vi "CBR_Player.vi"() -> ()   [LabVIEW 2012]
panel:
  out "Tiny Lines":string[](array[string])
  out "BotSpeak":string
  out "ComType":T1(ring)
  out "Reply":string
  out "error out":errorcluster
  out "text":string
  in  "Vireo":path=path "/Kim/Users/crogers/Documents/LabVIEW Data/LVVIAGenerated/Demo1.vi  2013-12-18 14-09-36.via"
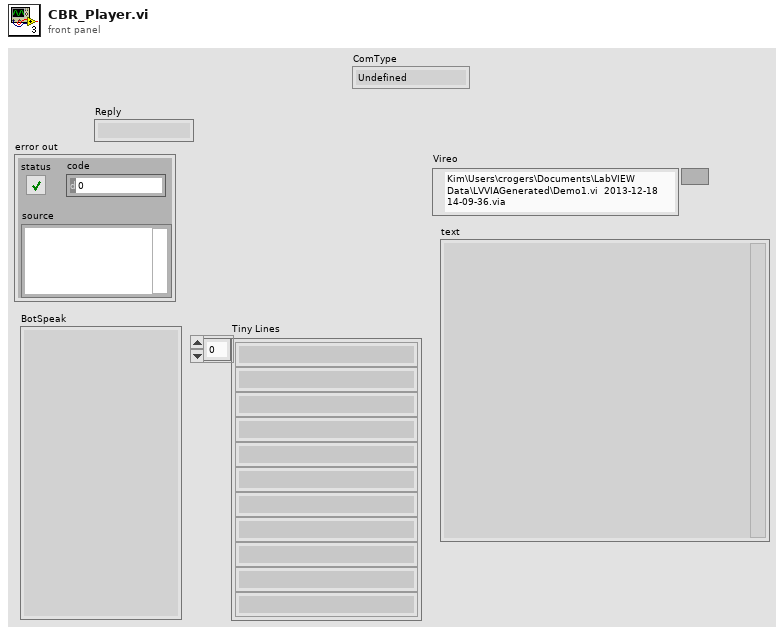
[diagram p1: front panel]
types:
  T1 = enum16{"Undefined", "HTTP", "Serial", "TCPIP", "Console"}
  T2 = typedef "BotSpeak_Control.ctl" = cluster{"Address":string, "Reply EOF":string, "Hardware":string, "Retries":i8, "Timeout":i32, "Open?":bool}
  T3 = typedef "BotSpeak.HardwareSpecs.ctl" = cluster{"Hardware Name":string, "Hardware URL":string, "ComType":enum16{"Undefined", "HTTP", "Serial", "TCPIP", "Console"}, "TCP Port":i32, "DefaultAddress":string, "Retries":i32, "Translate":enum16{"None", "Tiny", "URAPI"}, "MaxScriptSize":i32, "MaxVarNumber":i32, "StartupWait":i32, "Patience":i32, "Startup Patience":i32, "Hardware Help":string, "Com Protocol":string, "Translator":cluster{"BotSpeak CMD":string, "CMD out":string}[], "Init Code":string, "Variable Format":enum16{"INT", "FLOAT", "FIXED"}, "username":string, "password":string}
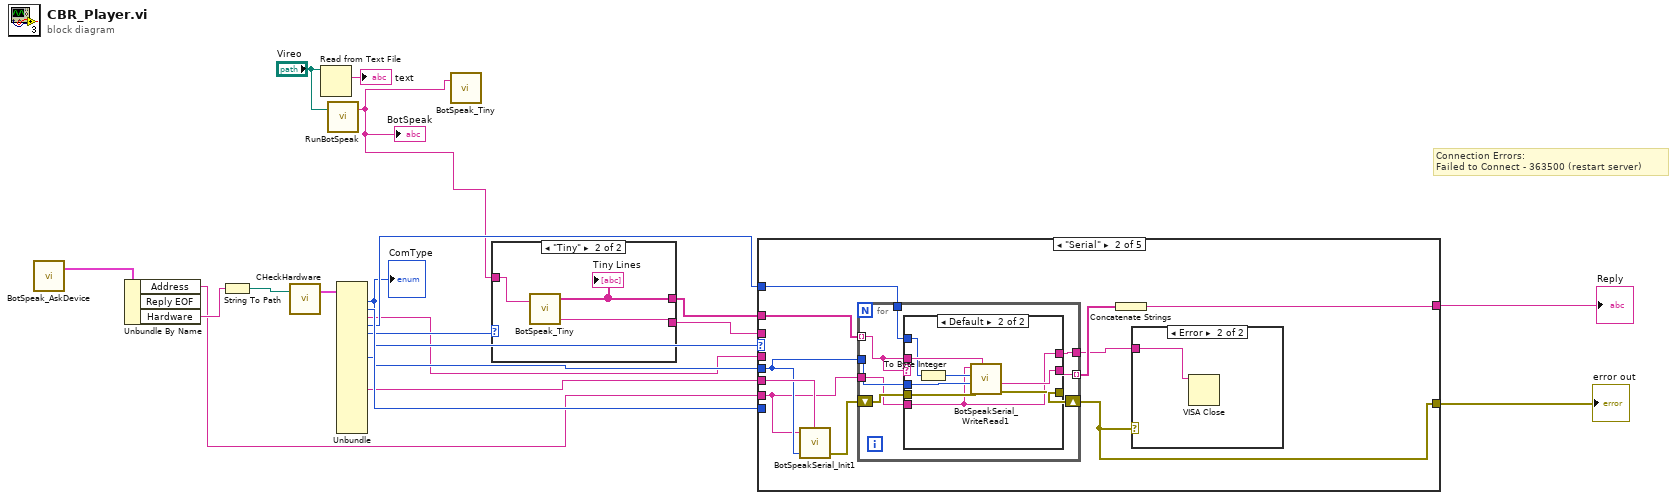
[diagram p0: block diagram]
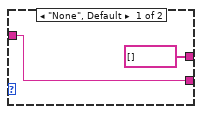
[diagram p2: hidden frame]
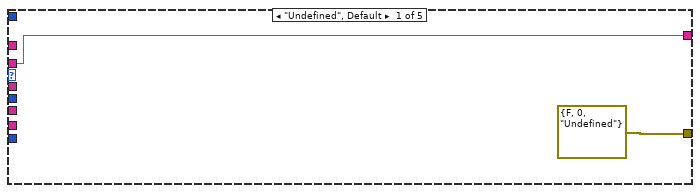
[diagram p3: hidden frame]
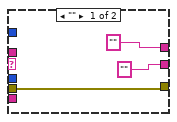
[diagram p4: hidden frame]
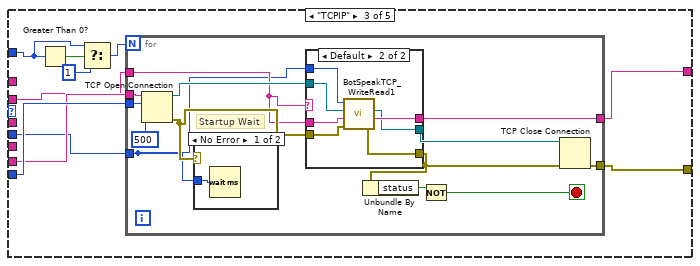
[diagram p6: hidden frame]
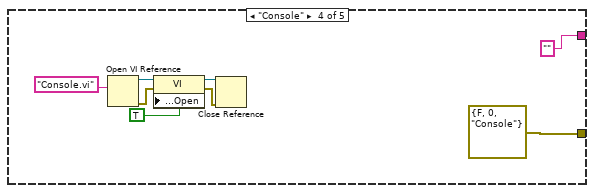
[diagram p9: hidden frame]
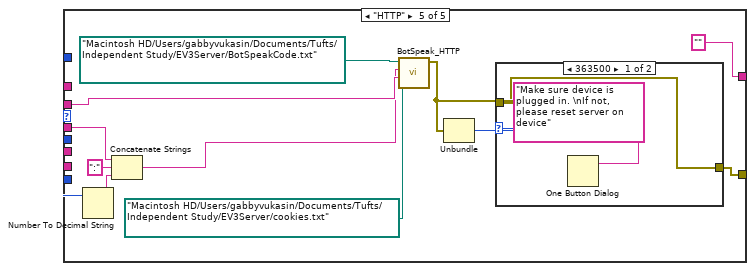
[diagram p10: hidden frame]
diagram:
  # "Connection Errors:\nFailed to Connect - 363500 (restart server)"
  n1 = call <userlib>:"BotSpeak_AskDevice.vi"() -> ("Bot Settings out"=w9:T2)  [unwired: 3 in]
  n2 = Unbundle By Name(w9) -> ("Address"=w5:string, "Hardware"=w8:string)  [unwired: 1 out]
  n3 = String To Path(string=w8) -> (path=w10:path)
  n4 = call <userlib>:"CHeckHardware.vi"("Hardware"=w10) -> ("HardwareSpecs"=w14:T3)  [unwired: 2 in]
  n5 = Read from Text File(file (use dialog)="Vireo") -> (text=→"text":string)  [unwired: 3 in, 3 out]
  n6 = call <userlib>:"RunBotSpeak.vi"("VIA"="Vireo") -> ("BotSpeak"=w1:string)  [unwired: 2 in]
  "BotSpeak" <- w1
  n7 = Unbundle(w14) -> ("ComType"=w13:T1, "TCP Port"=w19:i32, "DefaultAddress"=w4:string, "Retries"=w16:i32, "Translate"=w18:enum16{"None", "Tiny", "URAPI"}, "StartupWait"=w15:i32, "Com Protocol"=w12:string)  [unwired: 12 out]
  "ComType" <- w13
  n8 = call <userlib>:"BotSpeak_Tiny.vi"("URAPI"=w1) -> ()  [unwired: 1 in, 3 out]
  n9 = case shown="\"Tiny\"" w18 {
    tunnel: w1 -> [w21 w24]
    tunnel: [w21 w23] -> w17
    tunnel: [string[] [] ("Tiny Lines") w22] -> w6
    frame "None", Default {
    }
    frame "Tiny" {
      n10 = call <userlib>:"BotSpeak_Tiny.vi"("URAPI"=w24) -> ("URAPI  2"=w23:string, "Tiny Lines"=w22:string[])  [unwired: 1 in, 1 out]
      "Tiny Lines" <- w22
    }
  }
  n11 = case shown="\"Serial\"" w13 {
    tunnel: w17 -> [w25 _ w59 _ w108]
    tunnel: w5 -> [_ w31 w61 _ _]
    tunnel: w19 -> [_ _ w62 _ w106]
    tunnel: w16 -> [_ w34 w64 _ _]
    tunnel: w15 -> [_ w33 w60 _ _]
    tunnel: w12 -> [_ w36 _ _ _]
    tunnel: [errorcluster {"status"=FALSE, "code"=0, "source"="Undefined"} ("connection\nerror") w27 w58 errorcluster {"status"=FALSE, "code"=0, "source"="Console"} ("connection\nerror") w101] -> w11
    tunnel: [w25 w29 w57 "" ("Reply") "" ("Reply")] -> w7
    tunnel: w6 -> [_ w32 _ _ _]
    tunnel: w4 -> [_ _ _ _ w99]
    frame "Undefined", Default {
    }
    frame "Serial" {
      n12 = call <userlib>:"BotSpeakSerial_Init1.vi"("StartupWait"=w33, "Com Protocol"=w36, "Address"=w31) -> ("error out"=w35:errorcluster)  [unwired: 2 in]
      n13 = for {
        tunnel: w34 -> [w43]
        tunnel: w33 -> [w42]
        shift-right: [w41] -> w27
        shift-left: w35 -> [w44]
        tunnel: w32 -> [w40] mode=indexing
        tunnel: [w39] -> w30 mode=indexing
        tunnel: w31 -> [w38]
        tunnel: [w37] -> w28
        n14 = case shown="Default" w40 {
          tunnel: w44 -> [w47 w55]
          tunnel: [w47 w54] -> w41
          tunnel: w40 -> [_ w53]
          tunnel: w38 -> [_ w48]
          tunnel: w43 -> [_ w50]
          tunnel: w42 -> [_ w52]
          tunnel: ["" ("Reply") w49] -> w39
          tunnel: ["" ("DefaultAddress") w48] -> w37
          frame "" {
          }
          frame Default {
            n15 = To Byte Integer(number=w50) -> (8bit integer=w51:i8)
            n16 = call <userlib>:"BotSpeakSerial_WriteRead1.vi"("To Write"=w53, "error In"=w55, "Timeout"=w52, "Retries"=w51, "Address"=w48) -> ("error out"=w54:errorcluster, "Reply"=w49:string)  [unwired: 1 in, 1 out]
          }
        }
      }
      n17 = Concatenate Strings(w30) -> (w29:string)
      n18 = case shown="Error" w27 {
        tunnel: w28 -> [_ w56]
        frame No Error {
        }
        frame Error {
          n19 = VISA Close(VISA resource name=w56) -> ()  [unwired: 1 in, 1 out]
        }
      }
    }
    frame "TCPIP" {
      n20 = Greater Than 0?(x=w64) -> (x > 0?=w66:bool)
      n21 = Select(t=w64, s=w66, f=1) -> (s? t:f=w65:i32)
      n22 = for {
        N: w65 -> [_]
        tunnel: w62 -> [w79]
        tunnel: w61 -> [w77]
        tunnel: w60 -> [w71]
        tunnel: w59 -> [w74]
        tunnel: [w73] -> w57
        tunnel: [w70] -> w58
        stop <- w67 stop-if-true
        # "Startup Wait"
        n23 = TCP Open Connection(address=w77, remote port or service name=w79, timeout ms (60000)=500) -> (connection ID=w76:refnum<k5>, error out=w75:errorcluster)  [unwired: 2 in]
        n24 = case shown="No Error" w75 {
          tunnel: w71 -> [w90 _]
          frame No Error {
            n25 = Wait (ms)(milliseconds to wait=w90) -> ()  [unwired: 1 out]
          }
          frame Error {
          }
        }
        n26 = case shown="Default" w74 {
          tunnel: w76 -> [w81 w89]
          tunnel: w74 -> [w82 w88]
          tunnel: [w82 w87] -> w73
          tunnel: w75 -> [w80 w86]
          tunnel: [w81 w85] -> w72
          tunnel: [w80 w84] -> w69
          tunnel: w71 -> [_ w83]
          frame "" {
          }
          frame Default {
            n27 = call <userlib>:"BotSpeakTCP_WriteRead1.vi"("error in"=w86, "To Send"=w88, "connection ID"=w89, "Timeout"=w83) -> ("error out"=w84:errorcluster, "data out"=w87:string, "connection ID out"=w85:refnum<k5>)  [unwired: 1 in]
          }
        }
        n28 = Unbundle By Name(w69) -> ("status"=w68:bool)
        n29 = Not(x=w68) -> (.not. x?=w67:bool)
        n30 = TCP Close Connection(connection ID=w72, error in (no error)=w69) -> (error out=w70:errorcluster)  [unwired: 1 in, 1 out]
      }
    }
    frame "Console" {
      n31 = Open VI Reference(vi path="Console.vi" ("Status String")) -> (vi reference=w95:refnum<vi>, error out=w94:errorcluster)  [unwired: 5 in]
      n32 = property class="VI"(reference=w95, error in=w94, "Front Panel.Open"=TRUE ("Front Panel Window:Open")) -> (reference out=w91:refnum<vi>, error out=w92:errorcluster)
      n33 = Close Reference(reference=w91, error in (no error)=w92) -> ()  [unwired: 1 out]
    }
    frame "HTTP" {
      n34 = Number To Decimal String(number=w106) -> (decimal integer string=w105:string)  [unwired: 1 in]
      n35 = Concatenate Strings(w99, ":" ("string"), w105) -> (w100:string)
      n36 = call <userlib>:"BotSpeak_HTTP.vi"("BotSpeak File Name"=path "/Macintosh HD/Users/gabbyvukasin/Documents/Tufts/Independent Study/EV3Server/BotSpeakCode.txt", "URL"=w100, "BotSpeak Code"=w108, "cookie file"=path "/Macintosh HD/Users/gabbyvukasin/Documents/Tufts/Independent Study/EV3Server/cookies.txt") -> ("connection\nerror"=w102:errorcluster)  [unwired: 5 in, 1 out]
      n37 = Unbundle(w102) -> ("code"=w103:i32)  [unwired: 2 out]
      n38 = case shown="363500" w103 {
        tunnel: w102 -> [w111 w113]
        tunnel: [w111 w113] -> w101
        frame 363500 {
          n39 = One Button Dialog(message="Make sure device is plugged in. \nIf not, please reset server on device") -> ()  [unwired: 1 in, 1 out]
        }
        frame Default {
        }
      }
    }
  }
  "error out" <- w11
  "Reply" <- w7
